vi "Arcade Drive.vi"(9 "Max Output":dbl, 10 "Y Axis":dbl, 11 "X Axis":dbl) -> (2 "Left Motor Value":dbl, 3 "Right Motor Value":dbl)   [LabVIEW 2012]
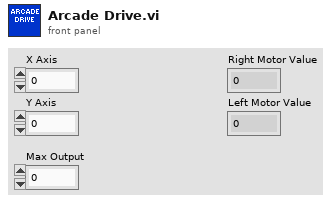
[diagram p1: front panel]
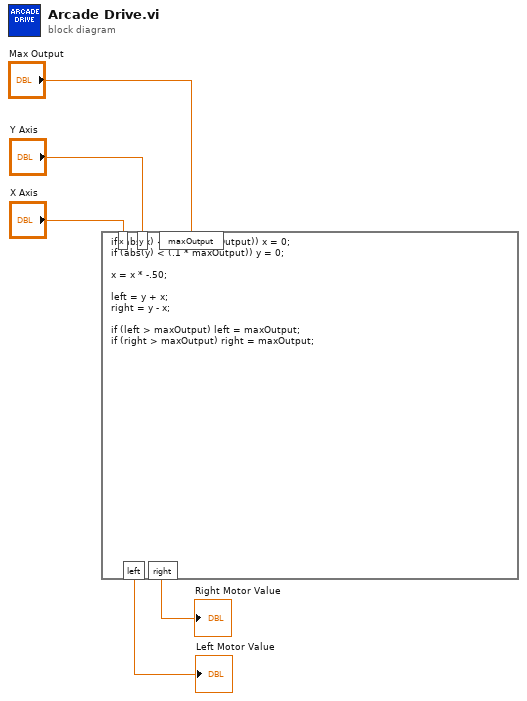
[diagram p0: block diagram]
diagram:
  n1 = formula code="if (abs(x) < (.15 * maxOutput)) x = 0;\nif (abs(y) < (.1 * maxOutput)) y = 0;\n\nx = x * -.50;\n\nleft = y + x;\nright = y - x;\n\nif (left > maxOutput) left = maxOutput;\nif (right > maxOutput) right = maxOutput;"("x"="X Axis", "y"="Y Axis", "maxOutput"="Max Output") -> ("left"=→"Left Motor Value":dbl, "right"=→"Right Motor Value":dbl)
